vi "RefChPowerP.vi"(0 "Pwr  P 4":refnum<vi>, 1 "Pwr  P 5":refnum<vi>, 2 "Pwr  P 6":refnum<vi>, 3 "Init_F":bool=TRUE, 4 "Pwr  P 7":refnum<vi>, 5 "Pwr  P 8":refnum<vi>, 6 "Pwr  P 9":refnum<vi>, 8 "Pwr  P 3":refnum<vi>, 9 "Pwr  P 10":refnum<vi>, 10 "Pwr  P 2":refnum<vi>, 11 "Pwr  P 11":refnum<vi>, 12 "Pwr  P 1":refnum<vi>, 13 "Pwr  P 12":refnum<vi>, 27 "error in":errorcluster) -> (7 "error out":errorcluster, 15 "Pwr  P1 out":refnum<vi>, 16 "Pwr  P12 out":refnum<vi>, 17 "Pwr  P2 out":refnum<vi>, 18 "Pwr  P11 out":refnum<vi>, 19 "Pwr  P3 out":refnum<vi>, 20 "Pwr  P10 out":refnum<vi>, 21 "Pwr  P9 out":refnum<vi>, 22 "Pwr  P8 out":refnum<vi>, 23 "Pwr  P7 out":refnum<vi>, 24 "Pwr  P6 out":refnum<vi>, 25 "Pwr  P5 out":refnum<vi>, 26 "Pwr  P4 out":refnum<vi>)   [LabVIEW 2017]
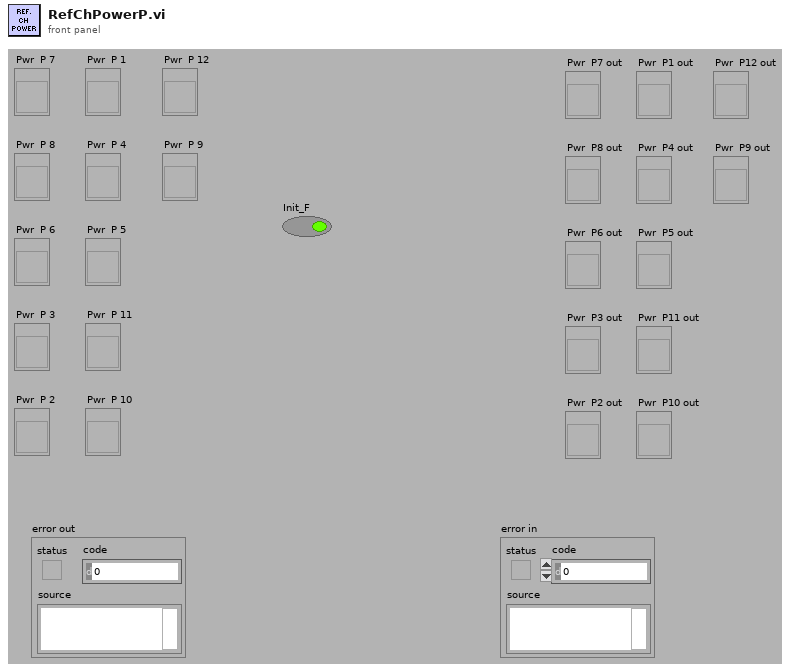
[diagram p1: front panel]
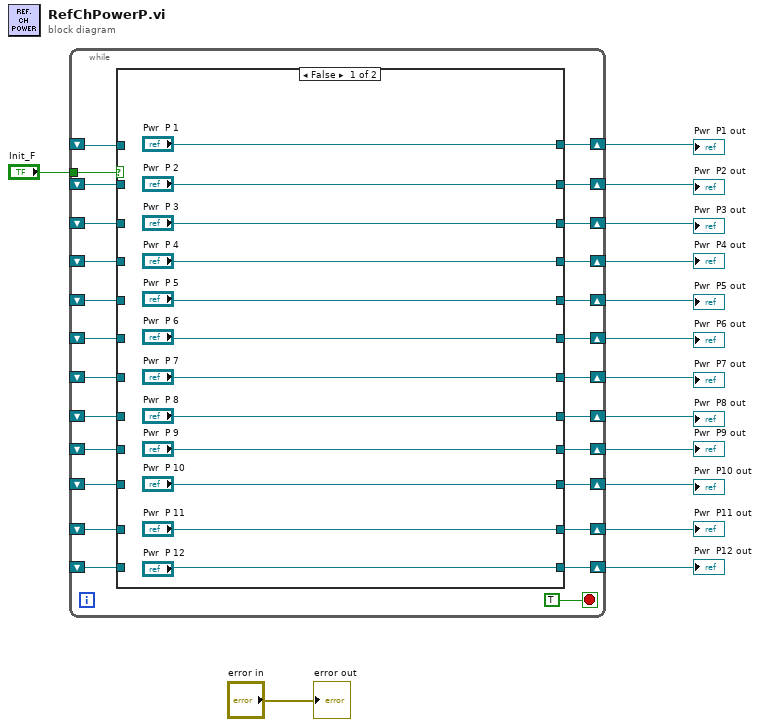
[diagram p0: block diagram]
diagram:
  n1 = while {
    shift-right: [w39] -> w12
    shift-left: _ -> [w38]
    tunnel: "Init_F" -> [w37]
    shift-right: [w36] -> w11
    shift-left: _ -> [w29]
    shift-right: [w35] -> w10
    shift-left: _ -> [w28]
    shift-right: [w34] -> w9
    shift-left: _ -> [w23]
    shift-right: [w33] -> w8
    shift-left: _ -> [w27]
    shift-right: [w32] -> w7
    shift-left: _ -> [w26]
    shift-right: [w31] -> w6
    shift-left: _ -> [w25]
    shift-right: [w30] -> w5
    shift-left: _ -> [w24]
    shift-right: [w22] -> w4
    shift-left: _ -> [w20]
    shift-right: [w21] -> w3
    shift-left: _ -> [w19]
    shift-right: [w18] -> w2
    shift-left: _ -> [w16]
    shift-right: [w17] -> w1
    shift-left: _ -> [w15]
    stop <- TRUE stop-if-true
    n2 = case shown="False" w37 {
      tunnel: ["Pwr  P 1" w64] -> w39
      tunnel: w38 -> [_ w64]
      tunnel: ["Pwr  P 2" w57] -> w36
      tunnel: ["Pwr  P 3" w58] -> w35
      tunnel: ["Pwr  P 4" w59] -> w34
      tunnel: ["Pwr  P 5" w60] -> w33
      tunnel: ["Pwr  P 6" w61] -> w32
      tunnel: ["Pwr  P 7" w62] -> w31
      tunnel: ["Pwr  P 8" w63] -> w30
      tunnel: w29 -> [_ w57]
      tunnel: w28 -> [_ w58]
      tunnel: w27 -> [_ w60]
      tunnel: w26 -> [_ w61]
      tunnel: w25 -> [_ w62]
      tunnel: w24 -> [_ w63]
      tunnel: w23 -> [_ w59]
      tunnel: ["Pwr  P 9" w56] -> w22
      tunnel: ["Pwr  P 10" w55] -> w21
      tunnel: w20 -> [_ w56]
      tunnel: w19 -> [_ w55]
      tunnel: ["Pwr  P 11" w54] -> w18
      tunnel: ["Pwr  P 12" w53] -> w17
      tunnel: w16 -> [_ w54]
      tunnel: w15 -> [_ w53]
      frame False {
      }
      frame True {
      }
    }
  }
  "Pwr  P1 out" <- w12
  "Pwr  P2 out" <- w11
  "Pwr  P3 out" <- w10
  "Pwr  P4 out" <- w9
  "Pwr  P5 out" <- w8
  "Pwr  P6 out" <- w7
  "Pwr  P7 out" <- w6
  "Pwr  P8 out" <- w5
  "Pwr  P9 out" <- w4
  "Pwr  P10 out" <- w3
  "Pwr  P11 out" <- w2
  "Pwr  P12 out" <- w1
  "error out" <- "error in"
